vi "Lab Panel V4.83.vi"() -> ()   [LabVIEW 2013] (continued)
                                n2698 = One Button Dialog(message=w4547) -> ()  [unwired: 1 in, 1 out]
                              }
                            }
                          }
                          frame #3 {
                            n2699 = Greater?(x=w4549, y=w4552) -> (0:w4551:bool)
                            n2700 = case shown="True" w4551 {
                              tunnel: [w4553 0] -> w4548
                              tunnel: w4549 -> [w4553 _]
                              tunnel: w4550 -> [_ w4554]
                              frame False {
                              }
                              frame True {
                                n2701 = Concatenate Strings("LA02-2 ", w4554) -> (w4557:string)
                                n2702 = One Button Dialog(message=w4557) -> ()  [unwired: 1 in, 1 out]
                              }
                            }
                          }
                          frame #4 {
                            n2703 = Greater?(x=w4559, y=w4562) -> (0:w4561:bool)
                            n2704 = case shown="True" w4561 {
                              tunnel: [w4563 0] -> w4558
                              tunnel: w4559 -> [w4563 _]
                              tunnel: w4560 -> [_ w4564]
                              frame False {
                              }
                              frame True {
                                n2705 = Concatenate Strings("LA03-1 ", w4564) -> (w4567:string)
                                n2706 = One Button Dialog(message=w4567) -> ()  [unwired: 1 in, 1 out]
                              }
                            }
                          }
                          frame #5 {
                            n2707 = Greater?(x=w4568, y=w4572) -> (0:w4571:bool)
                            n2708 = case shown="True" w4571 {
                              tunnel: [w4573 0] -> w4569
                              tunnel: w4568 -> [w4573 _]
                              tunnel: w4570 -> [_ w4574]
                              frame False {
                              }
                              frame True {
                                n2709 = Concatenate Strings("LA03-2 ", w4574) -> (w4577:string)
                                n2710 = One Button Dialog(message=w4577) -> ()  [unwired: 1 in, 1 out]
                              }
                            }
                          }
                          frame #6 {
                            n2711 = Greater?(x=w4579, y=w4582) -> (0:w4581:bool)
                            n2712 = case shown="True" w4581 {
                              tunnel: [w4583 0] -> w4578
                              tunnel: w4579 -> [w4583 _]
                              tunnel: w4580 -> [_ w4584]
                              frame False {
                              }
                              frame True {
                                n2713 = Concatenate Strings("LA04-1 ", w4584) -> (w4587:string)
                                n2714 = One Button Dialog(message=w4587) -> ()  [unwired: 1 in, 1 out]
                              }
                            }
                          }
                          frame #7 {
                            n2715 = Greater?(x=w4589, y=w4592) -> (0:w4591:bool)
                            n2716 = case shown="True" w4591 {
                              tunnel: [w4593 0] -> w4588
                              tunnel: w4589 -> [w4593 _]
                              tunnel: w4590 -> [_ w4594]
                              frame False {
                              }
                              frame True {
                                n2717 = Concatenate Strings("LA04-2 ", w4594) -> (w4597:string)
                                n2718 = One Button Dialog(message=w4597) -> ()  [unwired: 1 in, 1 out]
                              }
                            }
                          }
                          frame #8 {
                            n2719 = Greater?(x=w4599, y=w4602) -> (0:w4601:bool)
                            n2720 = case shown="True" w4601 {
                              tunnel: [w4603 0] -> w4598
                              tunnel: w4599 -> [w4603 _]
                              tunnel: w4600 -> [_ w4604]
                              frame False {
                              }
                              frame True {
                                n2721 = Concatenate Strings("LA05-1 ", w4604) -> (w4607:string)
                                n2722 = One Button Dialog(message=w4607) -> ()  [unwired: 1 in, 1 out]
                              }
                            }
                          }
                          frame #9 {
                            n2723 = Greater?(x=w4609, y=w4612) -> (0:w4611:bool)
                            n2724 = case shown="True" w4611 {
                              tunnel: [w4613 0] -> w4608
                              tunnel: w4609 -> [w4613 _]
                              tunnel: w4610 -> [_ w4614]
                              frame False {
                              }
                              frame True {
                                n2725 = Concatenate Strings("LA05-2 ", w4614) -> (w4617:string)
                                n2726 = One Button Dialog(message=w4617) -> ()  [unwired: 1 in, 1 out]
                              }
                            }
                          }
                        }
                        n2727 = Bundle By Name(cluster=w4516, "LAB01-1"=w4514, "LAB01-2"=w4512, "LAB02-1"=w4509, "LAB02-2"=w4506, "LAB03-1"=w4504, "LAB03-2"=w4503, "LAB04-1"=w4500, "LAB04-2"=w4498, "LAB05-1"=w4496, "LAB05-2"=w4494) -> (w4515:T7)
                        n2728 = local write "JIG RELAY CYCLES"(w4515) -> ()
                      }
                    }
                  }
                }
              }
            }
          }
          frame #19 {
            # "get temperature values"
            n2729 = local read "simulate"() -> (w4630:bool)
            n2730 = local read "Temp Test Cal"() -> (w4627:dbl)
            n2731 = stacked-sequence {
              tunnel: w4630 -> [_ w4686 w4731 w4776 w4821 w4866]
              tunnel: T12 {"1  (A) cal"=1.0, "1 (V) cal"=1.0, "1 (PF) cal"=1.0, "1 (TL) cal"=1.0, "1 (TN) cal"=1.0, "2 (A) cal"=1.0, "2 (V) cal"=1.0, "2 (PF) cal"=1.0, "2 (TL) cal"=1.0, "2 (TN) cal"=1.0} ("CAL LAB01") -> [_ w4685 w4730 w4775 w4820 w4865]
              tunnel: w4628 -> [_ w4683 _ _ _ _]
              tunnel: w4627 -> [_ w4679 w4729 w4774 w4819 w4864]
              tunnel: w4626 -> [_ w4674 _ _ _ _]
              tunnel: w4625 -> [_ _ w4720 _ _ _]
              tunnel: w4624 -> [_ _ w4719 _ _ _]
              tunnel: w4623 -> [_ _ _ w4765 _ _]
              tunnel: w4622 -> [_ _ _ w4764 _ _]
              tunnel: w4621 -> [_ _ _ _ w4810 _]
              tunnel: w4620 -> [_ _ _ _ w4809 _]
              tunnel: w4619 -> [_ _ _ _ _ w4855]
              tunnel: w4618 -> [_ _ _ _ _ w4854]
              frame #0 {
                n2732 = local read "Select COM port"() -> (w4635:refnum<visa-resource-name>)
                "COM port" <- w4635
                n2733 = local read "jig cycle"() -> (w4636:dbl)
                n2734 = local read "on loops"() -> (w4638:dbl)
                n2735 = global write "Global 1.vi" "tmp dly lps"("Temp Delay Lps") -> ()
                n2736 = global write "Global 1.vi" "dly value"("Temp Value") -> ()
                n2737 = Add(x=w4638, y=3) -> (x+y=w4639:dbl)
                n2738 = global write "Global 1.vi" "COM port"(w4635) -> ()
                n2739 = Equal?(x=w4636, y=w4639) -> (x = y?=w4632:bool)
                n2740 = local read "Temp Loops"() -> (w4631:dbl)
                n2741 = case shown="True" w4632 {
                  tunnel: w4631 -> [_ w4641]
                  frame False {
                  }
                  frame True {
                    n2742 = stacked-sequence {
                      tunnel: w4641 -> [w4644 w4672]
                      frame #0 {
                        n2743 = local read "simulate"() -> (w4642:bool)
                        n2744 = case shown="5" w4644 {
                          tunnel: 1.0 -> [_ w4649 w4651 w4657 w4661 w4666]
                          tunnel: w4642 -> [_ w4645 w4650 w4655 w4662 w4665]
                          frame 0, Default {
                          }
                          frame 1 {
                            w4647 = FALSE
                            n2745 = call "sub vi - GET ALL TEMP v5.vi"("LA01-EN"=TRUE, "simulate"=w4645, "LA02-EN"=w4647, "LA03-EN"=w4647, "LA04-EN"=w4647, "LA05-EN"=w4647, "Gen Cal Value"=w4649) -> ("LA01 TEMP"=w4646:T22)  [unwired: 3 in, 5 out]
                            n2746 = local write "LAB01 TEMP"(w4646) -> ()
                          }
                          frame 2 {
                            w4652 = FALSE
                            n2747 = call "sub vi - GET ALL TEMP v5.vi"("LA01-EN"=w4652, "simulate"=w4650, "LA02-EN"=TRUE, "LA03-EN"=w4652, "LA04-EN"=w4652, "LA05-EN"=w4652, "Gen Cal Value"=w4651) -> ("LA02 TEMP"=w4654:T22)  [unwired: 3 in, 5 out]
                            n2748 = local write "LAB02 TEMP"(w4654) -> ()
                          }
                          frame 3 {
                            w4658 = FALSE
                            n2749 = call "sub vi - GET ALL TEMP v5.vi"("LA01-EN"=w4658, "simulate"=w4655, "LA02-EN"=w4658, "LA03-EN"=TRUE, "LA04-EN"=w4658, "LA05-EN"=w4658, "Gen Cal Value"=w4657) -> ("LA03 TEMP"=w4656:T22)  [unwired: 3 in, 5 out]
                            n2750 = local write "LAB03 TEMP"(w4656) -> ()
                          }
                          frame 4 {
                            w4663 = FALSE
                            n2751 = call "sub vi - GET ALL TEMP v5.vi"("LA01-EN"=w4663, "simulate"=w4662, "LA02-EN"=w4663, "LA03-EN"=w4663, "LA04-EN"=TRUE, "LA05-EN"=w4663, "Gen Cal Value"=w4661) -> ("LA04 TEMP"=w4660:T22)  [unwired: 3 in, 5 out]
                            n2752 = local write "LAB04 TEMP"(w4660) -> ()
                          }
                          frame 5 {
                            w4668 = FALSE
                            n2753 = call "sub vi - GET ALL TEMP v5.vi"("LA01-EN"=w4668, "simulate"=w4665, "LA02-EN"=w4668, "LA03-EN"=w4668, "LA04-EN"=w4668, "LA05-EN"=TRUE, "Gen Cal Value"=w4666) -> ("LA05 TEMP"=w4667:T22)  [unwired: 3 in, 5 out]
                            n2754 = local write "LAB05 TEMP"(w4667) -> ()
                          }
                        }
                      }
                      frame #1 {
                        n2755 = Greater Or Equal?(x=w4672, y=5) -> (x >= y?=w4670:bool)
                        n2756 = case shown="True" w4670 {
                          frame False {
                          }
                          frame True {
                            n2757 = local write "Temp Loops"(0) -> ()
                          }
                        }
                      }
                    }
                    n2758 = local write "TEMP"(TRUE) -> ()
                  }
                }
              }
              frame #1 {
                n2759 = case shown="False" w4686 {
                  tunnel: [w4717 w4718] -> w4702
                  tunnel: w4685 -> [_ w4718]
                  frame False {
                    n2760 = local read "CAL LAB01"() -> (w4717:T12)
                  }
                  frame True {
                  }
                }
                n2761 = local read "LAB01 TEMP"() -> (w4692:T11)
                n2762 = local read "TEMP LA01"() -> (w4693:T8)
                n2763 = call "sub vi - temperature delay v2.vi"("temp values IN"=w4693, "temp signals"=w4692) -> ("T2-N"=w4688:dbl, "T2-L"=w4689:dbl, "T1-N"=w4690:dbl, "T1-L"=w4691:dbl, "temp values OUT"=w4687:T39)  [unwired: 5 in]
                n2764 = Unbundle By Name(w4702) -> ("1 (TL) cal"=w4697:dbl, "1 (TN) cal"=w4696:dbl, "2 (TL) cal"=w4695:dbl, "2 (TN) cal"=w4694:dbl)  [unwired: 6 out]
                n2765 = local write "TEMP LA01"(w4687) -> ()
                n2766 = Multiply(x=w4691, y=w4697) -> (x*y=w4684:dbl)
                n2767 = Multiply(x=w4690, y=w4696) -> (x*y=w4681:dbl)
                n2768 = Multiply(x=w4689, y=w4695) -> (x*y=w4678:dbl)
                n2769 = Multiply(x=w4688, y=w4694) -> (x*y=w4677:dbl)
                n2770 = case shown="True" w4683 {
                  tunnel: w4684 -> [w4711 w4716]
                  tunnel: w4679 -> [_ w4714]
                  tunnel: [w4711 w4715] -> w4682
                  tunnel: w4681 -> [w4710 w4713]
                  tunnel: [w4710 w4712] -> w4680
                  frame False {
                  }
                  frame True {
                    n2771 = Multiply(x=w4714, y=w4713) -> (x*y=w4712:dbl)
                    n2772 = Multiply(x=w4714, y=w4716) -> (x*y=w4715:dbl)
                  }
                }
                n2773 = case shown="True" w4674 {
                  tunnel: w4678 -> [w4704 w4709]
                  tunnel: w4679 -> [_ w4707]
                  tunnel: [w4704 w4708] -> w4676
                  tunnel: w4677 -> [w4703 w4706]
                  tunnel: [w4703 w4705] -> w4675
                  frame False {
                  }
                  frame True {
                    n2774 = Multiply(x=w4707, y=w4706) -> (x*y=w4705:dbl)
                    n2775 = Multiply(x=w4707, y=w4709) -> (x*y=w4708:dbl)
                  }
                }
                n2776 = local read "SIG LAB01-2"() -> (w4699:T2)
                n2777 = local read "SIG LAB01-1"() -> (w4701:T2)
                n2778 = Bundle By Name(cluster=w4701, "Tmp Live"=w4682, "Tmp Neut"=w4680) -> (w4700:T2)
                n2779 = Bundle By Name(cluster=w4699, "Tmp Live"=w4676, "Tmp Neut"=w4675) -> (w4698:T2)
                n2780 = local write "SIG LAB01-1"(w4700) -> ()
                n2781 = local write "SIG LAB01-2"(w4698) -> ()
              }
              frame #2 {
                n2782 = case shown="True" w4731 {
                  tunnel: [w4762 w4763] -> w4747
                  tunnel: w4730 -> [_ w4763]
                  frame False {
                    n2783 = local read "CAL LAB02"() -> (w4762:T13)
                  }
                  frame True {
                  }
                }
                n2784 = local read "LAB02 TEMP"() -> (w4738:T11)
                n2785 = local read "TEMP LA02"() -> (w4737:T8)
                n2786 = call "sub vi - temperature delay v2.vi"("temp values IN"=w4737, "temp signals"=w4738) -> ("T2-N"=w4732:dbl, "T2-L"=w4733:dbl, "T1-N"=w4734:dbl, "T1-L"=w4735:dbl, "temp values OUT"=w4736:T39)  [unwired: 5 in]
                n2787 = Unbundle By Name(w4747) -> ("1 (TL) cal"=w4742:dbl, "1 (TN) cal"=w4741:dbl, "2 (TL) cal"=w4740:dbl, "2 (TN) cal"=w4739:dbl)  [unwired: 6 out]
                n2788 = local write "TEMP LA02"(w4736) -> ()
                n2789 = Multiply(x=w4735, y=w4742) -> (x*y=w4728:dbl)
                n2790 = Multiply(x=w4734, y=w4741) -> (x*y=w4727:dbl)
                n2791 = Multiply(x=w4733, y=w4740) -> (x*y=w4724:dbl)
                n2792 = Multiply(x=w4732, y=w4739) -> (x*y=w4723:dbl)
                n2793 = case shown="True" w4720 {
                  tunnel: w4728 -> [w4756 w4761]
                  tunnel: w4729 -> [_ w4759]
                  tunnel: [w4756 w4760] -> w4726
                  tunnel: w4727 -> [w4755 w4758]
                  tunnel: [w4755 w4757] -> w4725
                  frame False {
                  }
                  frame True {
                    n2794 = Multiply(x=w4759, y=w4758) -> (x*y=w4757:dbl)
                    n2795 = Multiply(x=w4759, y=w4761) -> (x*y=w4760:dbl)
                  }
                }
                n2796 = case shown="True" w4719 {
                  tunnel: w4724 -> [w4749 w4754]
                  tunnel: w4729 -> [_ w4752]
                  tunnel: [w4749 w4753] -> w4722
                  tunnel: w4723 -> [w4748 w4751]
                  tunnel: [w4748 w4750] -> w4721
                  frame False {
                  }
                  frame True {
                    n2797 = Multiply(x=w4752, y=w4751) -> (x*y=w4750:dbl)
                    n2798 = Multiply(x=w4752, y=w4754) -> (x*y=w4753:dbl)
                  }
                }
                n2799 = local read "SIG LAB02-2"() -> (w4744:T2)
                n2800 = local read "SIG LAB02-1"() -> (w4746:T2)
                n2801 = Bundle By Name(cluster=w4746, "Tmp Live"=w4726, "Tmp Neut"=w4725) -> (w4745:T2)
                n2802 = Bundle By Name(cluster=w4744, "Tmp Live"=w4722, "Tmp Neut"=w4721) -> (w4743:T2)
                n2803 = local write "SIG LAB02-1"(w4745) -> ()
                n2804 = local write "SIG LAB02-2"(w4743) -> ()
              }
              frame #3 {
                n2805 = case shown="False" w4776 {
                  tunnel: [w4807 w4808] -> w4792
                  tunnel: w4775 -> [_ w4808]
                  frame False {
                    n2806 = local read "CAL LAB03"() -> (w4807:T12)
                  }
                  frame True {
                  }
                }
                n2807 = local read "TEMP LA03"() -> (w4782:T8)
                n2808 = local read "LAB03 TEMP"() -> (w4783:T11)
                n2809 = call "sub vi - temperature delay v2.vi"("temp values IN"=w4782, "temp signals"=w4783) -> ("T2-N"=w4777:dbl, "T2-L"=w4778:dbl, "T1-N"=w4779:dbl, "T1-L"=w4780:dbl, "temp values OUT"=w4781:T39)  [unwired: 5 in]
                n2810 = Unbundle By Name(w4792) -> ("1 (TL) cal"=w4787:dbl, "1 (TN) cal"=w4786:dbl, "2 (TL) cal"=w4785:dbl, "2 (TN) cal"=w4784:dbl)  [unwired: 6 out]
                n2811 = local write "TEMP LA03"(w4781) -> ()
                n2812 = Multiply(x=w4780, y=w4787) -> (x*y=w4773:dbl)
                n2813 = Multiply(x=w4779, y=w4786) -> (x*y=w4772:dbl)
                n2814 = Multiply(x=w4778, y=w4785) -> (x*y=w4769:dbl)
                n2815 = Multiply(x=w4777, y=w4784) -> (x*y=w4768:dbl)
                n2816 = case shown="True" w4764 {
                  tunnel: w4769 -> [w4794 w4799]
                  tunnel: w4774 -> [_ w4797]
                  tunnel: [w4794 w4798] -> w4767
                  tunnel: w4768 -> [w4793 w4796]
                  tunnel: [w4793 w4795] -> w4766
                  frame False {
                  }
                  frame True {
                    n2817 = Multiply(x=w4797, y=w4796) -> (x*y=w4795:dbl)
                    n2818 = Multiply(x=w4797, y=w4799) -> (x*y=w4798:dbl)
                  }
                }
                n2819 = case shown="True" w4765 {
                  tunnel: w4773 -> [w4801 w4806]
                  tunnel: w4774 -> [_ w4804]
                  tunnel: [w4801 w4805] -> w4771
                  tunnel: w4772 -> [w4800 w4803]
                  tunnel: [w4800 w4802] -> w4770
                  frame False {
                  }
                  frame True {
                    n2820 = Multiply(x=w4804, y=w4803) -> (x*y=w4802:dbl)
                    n2821 = Multiply(x=w4804, y=w4806) -> (x*y=w4805:dbl)
                  }
                }
                n2822 = local read "SIG LAB03-2"() -> (w4789:T2)
                n2823 = local read "SIG LAB03-1"() -> (w4791:T2)
                n2824 = Bundle By Name(cluster=w4791, "Tmp Live"=w4771, "Tmp Neut"=w4770) -> (w4790:T2)
                n2825 = Bundle By Name(cluster=w4789, "Tmp Live"=w4767, "Tmp Neut"=w4766) -> (w4788:T2)
                n2826 = local write "SIG LAB03-1"(w4790) -> ()
                n2827 = local write "SIG LAB03-2"(w4788) -> ()
              }
              frame #4 {
                n2828 = case shown="False" w4821 {
                  tunnel: [w4852 w4853] -> w4837
                  tunnel: w4820 -> [_ w4853]
                  frame False {
                    n2829 = local read "CAL LAB04"() -> (w4852:T12)
                  }
                  frame True {
                  }
                }
                n2830 = local read "LAB04 TEMP"() -> (w4827:T11)
                n2831 = local read "TEMP LA04"() -> (w4828:T8)
                n2832 = call "sub vi - temperature delay v2.vi"("temp values IN"=w4828, "temp signals"=w4827) -> ("T2-N"=w4822:dbl, "T2-L"=w4823:dbl, "T1-N"=w4824:dbl, "T1-L"=w4825:dbl, "temp values OUT"=w4826:T39)  [unwired: 5 in]
                n2833 = Unbundle By Name(w4837) -> ("1 (TL) cal"=w4832:dbl, "1 (TN) cal"=w4831:dbl, "2 (TL) cal"=w4830:dbl, "2 (TN) cal"=w4829:dbl)  [unwired: 6 out]
                n2834 = local write "TEMP LA04"(w4826) -> ()
                n2835 = Multiply(x=w4825, y=w4832) -> (x*y=w4818:dbl)
                n2836 = Multiply(x=w4824, y=w4831) -> (x*y=w4817:dbl)
                n2837 = Multiply(x=w4823, y=w4830) -> (x*y=w4814:dbl)
                n2838 = Multiply(x=w4822, y=w4829) -> (x*y=w4813:dbl)
                n2839 = case shown="True" w4809 {
                  tunnel: w4814 -> [w4839 w4844]
                  tunnel: w4819 -> [_ w4842]
                  tunnel: [w4839 w4843] -> w4812
                  tunnel: w4813 -> [w4838 w4841]
                  tunnel: [w4838 w4840] -> w4811
                  frame False {
                  }
                  frame True {
                    n2840 = Multiply(x=w4842, y=w4841) -> (x*y=w4840:dbl)
                    n2841 = Multiply(x=w4842, y=w4844) -> (x*y=w4843:dbl)
                  }
                }
                n2842 = case shown="True" w4810 {
                  tunnel: w4818 -> [w4846 w4851]
                  tunnel: w4819 -> [_ w4849]
                  tunnel: [w4846 w4850] -> w4816
                  tunnel: w4817 -> [w4845 w4848]
                  tunnel: [w4845 w4847] -> w4815
                  frame False {
                  }
                  frame True {
                    n2843 = Multiply(x=w4849, y=w4848) -> (x*y=w4847:dbl)
                    n2844 = Multiply(x=w4849, y=w4851) -> (x*y=w4850:dbl)
                  }
                }
                n2845 = local read "SIG LAB04-2"() -> (w4834:T2)
                n2846 = local read "SIG LAB04-1"() -> (w4836:T2)
                n2847 = Bundle By Name(cluster=w4836, "Tmp Live"=w4816, "Tmp Neut"=w4815) -> (w4835:T2)
                n2848 = Bundle By Name(cluster=w4834, "Tmp Live"=w4812, "Tmp Neut"=w4811) -> (w4833:T2)
                n2849 = local write "SIG LAB04-1"(w4835) -> ()
                n2850 = local write "SIG LAB04-2"(w4833) -> ()
              }
              frame #5 {
                n2851 = case shown="False" w4866 {
                  tunnel: [w4897 w4898] -> w4882
                  tunnel: w4865 -> [_ w4898]
                  frame False {
                    n2852 = local read "CAL LAB05"() -> (w4897:T12)
                  }
                  frame True {
                  }
                }
                n2853 = local read "LAB05 TEMP"() -> (w4872:T11)
                n2854 = local read "TEMP LA05"() -> (w4873:T8)
                n2855 = call "sub vi - temperature delay v2.vi"("temp values IN"=w4873, "temp signals"=w4872) -> ("T2-N"=w4868:dbl, "T2-L"=w4869:dbl, "T1-N"=w4870:dbl, "T1-L"=w4871:dbl, "temp values OUT"=w4867:T39)  [unwired: 5 in]
                n2856 = local write "TEMP LA05"(w4867) -> ()
                n2857 = Unbundle By Name(w4882) -> ("1 (TL) cal"=w4874:dbl, "1 (TN) cal"=w4877:dbl, "2 (TL) cal"=w4876:dbl, "2 (TN) cal"=w4875:dbl)  [unwired: 6 out]
                n2858 = Multiply(x=w4871, y=w4874) -> (x*y=w4863:dbl)
                n2859 = Multiply(x=w4870, y=w4877) -> (x*y=w4862:dbl)
                n2860 = Multiply(x=w4869, y=w4876) -> (x*y=w4859:dbl)
                n2861 = Multiply(x=w4868, y=w4875) -> (x*y=w4858:dbl)
                n2862 = case shown="True" w4854 {
                  tunnel: w4859 -> [w4884 w4889]
                  tunnel: w4864 -> [_ w4887]
                  tunnel: [w4884 w4888] -> w4857
                  tunnel: w4858 -> [w4883 w4886]
                  tunnel: [w4883 w4885] -> w4856
                  frame False {
                  }
                  frame True {
                    n2863 = Multiply(x=w4887, y=w4886) -> (x*y=w4885:dbl)
                    n2864 = Multiply(x=w4887, y=w4889) -> (x*y=w4888:dbl)
                  }
                }
                n2865 = case shown="True" w4855 {
                  tunnel: w4863 -> [w4891 w4896]
                  tunnel: w4864 -> [_ w4894]
                  tunnel: [w4891 w4895] -> w4861
                  tunnel: w4862 -> [w4890 w4893]
                  tunnel: [w4890 w4892] -> w4860
                  frame False {
                  }
                  frame True {
                    n2866 = Multiply(x=w4894, y=w4893) -> (x*y=w4892:dbl)
                    n2867 = Multiply(x=w4894, y=w4896) -> (x*y=w4895:dbl)
                  }
                }
                n2868 = local read "SIG LAB05-1"() -> (w4881:T2)
                n2869 = Bundle By Name(cluster=w4881, "Tmp Live"=w4861, "Tmp Neut"=w4860) -> (w4880:T2)
                n2870 = local read "SIG LAB05-2"() -> (w4879:T2)
                n2871 = Bundle By Name(cluster=w4879, "Tmp Live"=w4857, "Tmp Neut"=w4856) -> (w4878:T2)
                n2872 = local write "SIG LAB05-1"(w4880) -> ()
                n2873 = local write "SIG LAB05-2"(w4878) -> ()
              }
            }
          }
          frame #20 {
            # "write data to display panel"
            n2874 = global write "Global display 1.vi" "TEST 5-2"(w4913) -> ()
            n2875 = global write "Global display 1.vi" "TEST 4-2"(w4915) -> ()
            n2876 = global write "Global display 1.vi" "TEST 1-2"(w4921) -> ()
            n2877 = global write "Global display 1.vi" "TEST 3-1"(w4918) -> ()
            n2878 = global write "Global display 1.vi" "TEST 5-1"(w4914) -> ()
            n2879 = global write "Global display 1.vi" "TEST 1-1"(w4922) -> ()
            n2880 = global write "Global display 1.vi" "TEST 3-2"(w4917) -> ()
            n2881 = global write "Global display 1.vi" "TEST 4-1"(w4916) -> ()
            n2882 = global write "Global display 1.vi" "TEST 2-2"(w4919) -> ()
            n2883 = global write "Global display 1.vi" "TEST 2-1"(w4920) -> ()
            n2884 = global read "Global display 3.vi" "log 1-1"() -> (→"LOG LAB01-1":string)
            n2885 = global read "Global display 3.vi" "log 3-1"() -> (→"LOG LAB03-1":string)
            n2886 = global read "Global display 3.vi" "log 1-2"() -> (→"LOG LAB01-2":string)
            n2887 = property on="Tab Control 2" class="TabCtl (strict)"() -> ("Pages"=w4912:refnum<vi>[])  [unwired: 2 in, 2 out]
            n2888 = global read "Global display 3.vi" "log 2-1"() -> (→"LOG LAB02-1":string)
            n2889 = global read "Global display 3.vi" "log 2-2"() -> (→"LOG LAB02-2":string)
            n2890 = global read "Global display 3.vi" "log 4-2"() -> (→"LOG LAB04-2":string)
            n2891 = global read "Global display 3.vi" "log 5-2"() -> (→"LOG LAB05-2":string)
            n2892 = global read "Global display 3.vi" "log 5-1"() -> (→"LOG LAB05-1":string)
            n2893 = global read "Global display 3.vi" "log 4-1"() -> (→"LOG LAB04-1":string)
            n2894 = global read "Global display 3.vi" "log 3-2"() -> (→"LOG LAB03-2":string)
            n2895 = Index Array(array=w4912, index=9) -> (element=w4910:refnum<vi>)
            n2896 = property class="Page"(reference=w4910) -> ("PageVis"=w4909:bool)  [unwired: 1 in, 2 out]
            n2897 = global write "Global display 3.vi" "admin"(w4909) -> ()
            n2898 = local read "O/I  LAB05-2"() -> (w4963:bool)
            n2899 = local read "O/I  LAB05-1"() -> (w4964:bool)
            n2900 = local read "O/I  LAB03-2"() -> (w4967:bool)
            n2901 = local read "O/I  LAB04-2"() -> (w4965:bool)
            n2902 = local read "O/I  LAB04-1"() -> (w4966:bool)
            n2903 = local read "O/I  LAB03-1"() -> (w4968:bool)
            n2904 = local read "O/I  LAB01-2"() -> (w4971:bool)
            n2905 = local read "O/I  LAB01-1"() -> (w4972:bool)
            n2906 = local read "O/I  LAB02-1"() -> (w4970:bool)
            n2907 = local read "O/I  LAB02-2"() -> (w4969:bool)
            n2908 = global write "Global display 1.vi" "5-2 O/F"(w4963) -> ()
            n2909 = global write "Global display 1.vi" "5-1 O/F"(w4964) -> ()
            n2910 = global write "Global display 1.vi" "4-1 O/F"(w4966) -> ()
            n2911 = global write "Global display 1.vi" "4-2 O/F"(w4965) -> ()
            n2912 = global write "Global display 1.vi" "3-2 O/F"(w4967) -> ()
            n2913 = global write "Global display 1.vi" "3-1 O/F"(w4968) -> ()
            n2914 = global write "Global display 1.vi" "2-2 O/F"(w4969) -> ()
            n2915 = global write "Global display 1.vi" "2-1 O/F"(w4970) -> ()
            n2916 = global write "Global display 1.vi" "1-2 O/F"(w4971) -> ()
            n2917 = global write "Global display 1.vi" "1-1 O/F"(w4972) -> ()
            n2918 = local read "run lab05-2"() -> (w4953:bool)
            n2919 = local read "run lab04-1"() -> (w4956:bool)
            n2920 = local read "run lab04-2"() -> (w4955:bool)
            n2921 = local read "run lab05-1"() -> (w4954:bool)
            n2922 = local read "run lab03-2"() -> (w4957:bool)
            n2923 = local read "run lab02-1"() -> (w4960:bool)
            n2924 = local read "run lab03-1"() -> (w4958:bool)
            n2925 = local read "run lab01-2"() -> (w4961:bool)
            n2926 = local read "run lab02-2"() -> (w4959:bool)
            n2927 = local read "run lab01-1"() -> (w4962:bool)
            n2928 = global write "Global display 1.vi" "5-2 R/S"(w4953) -> ()
            n2929 = global write "Global display 1.vi" "5-1 R/S"(w4954) -> ()
            n2930 = global write "Global display 1.vi" "4-2 R/S"(w4955) -> ()
            n2931 = global write "Global display 1.vi" "4-1 R/S"(w4956) -> ()
            n2932 = global write "Global display 1.vi" "3-2 R/S"(w4957) -> ()
            n2933 = global write "Global display 1.vi" "1-2 R/S"(w4961) -> ()
            n2934 = global write "Global display 1.vi" "2-1 R/S"(w4960) -> ()
            n2935 = global write "Global display 1.vi" "3-1 R/S"(w4958) -> ()
            n2936 = global write "Global display 1.vi" "2-2 R/S"(w4959) -> ()
            n2937 = global write "Global display 1.vi" "1-1 R/S"(w4962) -> ()
            n2938 = local read "DISP LAB04-2"() -> (w4945:T4)
            n2939 = local read "DISP LAB05-1"() -> (w4944:T4)
            n2940 = local read "DISP LAB04-1"() -> (w4946:T4)
            n2941 = local read "DISP LAB05-2"() -> (w4943:T4)
            n2942 = local read "DISP LAB03-1"() -> (w4948:T4)
            n2943 = local read "DISP LAB03-2"() -> (w4947:T4)
            n2944 = local read "DISP LAB01-2"() -> (w4951:T4)
            n2945 = local read "DISP LAB02-1"() -> (w4950:T4)
            n2946 = local read "DISP LAB02-2"() -> (w4949:T4)
            n2947 = local read "DISP LAB01-1"() -> (w4952:T4)
            n2948 = global write "Global display 2.vi" "DISP LAB05-1"(w4944) -> ()
            n2949 = global write "Global display 2.vi" "DISP LAB05-2"(w4943) -> ()
            n2950 = global write "Global display 2.vi" "DISP LAB04-2"(w4945) -> ()
            n2951 = global write "Global display 2.vi" "DISP LAB02-1"(w4950) -> ()
            n2952 = global write "Global display 2.vi" "DISP LAB02-2"(w4949) -> ()
            n2953 = global write "Global display 2.vi" "DISP LAB04-1"(w4946) -> ()
            n2954 = global write "Global display 2.vi" "DISP LAB01-2"(w4951) -> ()
            n2955 = global write "Global display 2.vi" "DISP LAB01-1"(w4952) -> ()
            n2956 = global write "Global display 2.vi" "DISP LAB03-1"(w4948) -> ()
            n2957 = global write "Global display 2.vi" "DISP LAB03-2"(w4947) -> ()
            n2958 = local read "SET LAB05-2"() -> (w4933:T5)
            n2959 = local read "SET LAB05-1"() -> (w4934:T5)
            n2960 = local read "SET LAB04-1"() -> (w4936:T5)
            n2961 = local read "SET LAB04-2"() -> (w4935:T5)
            n2962 = local read "SET LAB03-1"() -> (w4938:T5)
            n2963 = local read "SET LAB03-2"() -> (w4937:T5)
            n2964 = local read "SET LAB02-2"() -> (w4939:T5)
            n2965 = local read "SET LAB01-2"() -> (w4941:T5)
            n2966 = local read "SET LAB02-1"() -> (w4940:T5)
            n2967 = local read "SET LAB01-1"() -> (w4942:T5)
            n2968 = global write "Global display 2.vi" "SET LAB05-2"(w4933) -> ()
            n2969 = global write "Global display 2.vi" "SET LAB05-1"(w4934) -> ()
            n2970 = global write "Global display 2.vi" "SET LAB04-1"(w4936) -> ()
            n2971 = global write "Global display 2.vi" "SET LAB04-2"(w4935) -> ()
            n2972 = global write "Global display 2.vi" "SET LAB03-2"(w4937) -> ()
            n2973 = global write "Global display 2.vi" "SET LAB02-2"(w4939) -> ()
            n2974 = global write "Global display 2.vi" "SET LAB03-1"(w4938) -> ()
            n2975 = global write "Global display 2.vi" "SET LAB01-2"(w4941) -> ()
            n2976 = global write "Global display 2.vi" "SET LAB01-1"(w4942) -> ()
            n2977 = global write "Global display 2.vi" "SET LAB02-1"(w4940) -> ()
            n2978 = local read "RESULT LAB01-1"() -> (w4932:bool)
            n2979 = local read "RESULT LAB03-2"() -> (w4927:bool)
            n2980 = local read "RESULT LAB04-1"() -> (w4926:bool)
            n2981 = local read "RESULT LAB04-2"() -> (w4925:bool)
            n2982 = local read "RESULT LAB02-2"() -> (w4929:bool)
            n2983 = local read "RESULT LAB01-2"() -> (w4931:bool)
            n2984 = local read "RESULT LAB02-1"() -> (w4930:bool)
            n2985 = local read "RESULT LAB03-1"() -> (w4928:bool)
            n2986 = local read "RESULT LAB05-1"() -> (w4924:bool)
            n2987 = local read "RESULT LAB05-2"() -> (w4923:bool)
            n2988 = global write "Global display 2.vi" "RESULT LAB05-1"(w4924) -> ()
            n2989 = global write "Global display 2.vi" "RESULT LAB01-2"(w4931) -> ()
            n2990 = global write "Global display 2.vi" "RESULT LAB03-2"(w4927) -> ()
            n2991 = global write "Global display 2.vi" "RESULT LAB04-1"(w4926) -> ()
            n2992 = global write "Global display 2.vi" "RESULT LAB04-2"(w4925) -> ()
            n2993 = global write "Global display 2.vi" "RESULT LAB05-2"(w4923) -> ()
            n2994 = global write "Global display 2.vi" "RESULT LAB03-1"(w4928) -> ()
            n2995 = global write "Global display 2.vi" "RESULT LAB02-1"(w4930) -> ()
            n2996 = global write "Global display 2.vi" "RESULT LAB02-2"(w4929) -> ()
            n2997 = global write "Global display 2.vi" "RESULT LAB01-1"(w4932) -> ()
          }
          frame #21 {
            # "end main and display program"
            n2998 = Quit LabVIEW(quit? (T)="stop all") -> ()
            n2999 = global write "Global display 1.vi" "stop disp"("stop all") -> ()
          }
        }
        n3000 = node-c288() -> ()  [unwired: 1 in, 1 out]
        "loops" <- w287
      }
      n3001 = node-c288(w264) -> ()  [unwired: 1 out]
    }
  }
